vi "CheckingLimits.vi"(7 "References":T1, 10 "Limits":dbl[](array[numeric]), 11 "Data":dbl) -> (3 "Color":u32)   [LabVIEW 2019]
uses:
  TypeDef/#TypeDef_References.ctl
  TypeDef/#TypeDef_Buttons.ctl
  TypeDef/#TypeDef_ReferencesMeassurementProp.ctl
  TypeDef/#TypeDef_ReferencesArchiveProp.ctl
  TypeDef/#TypeDef_Lists.ctl
  TypeDef/#TypeDef_MeasProp.ctl
  TypeDef/#TypeDef_OpProp.ctl
  TypeDef/#TypeDef_Enum_ModeOp.ctl
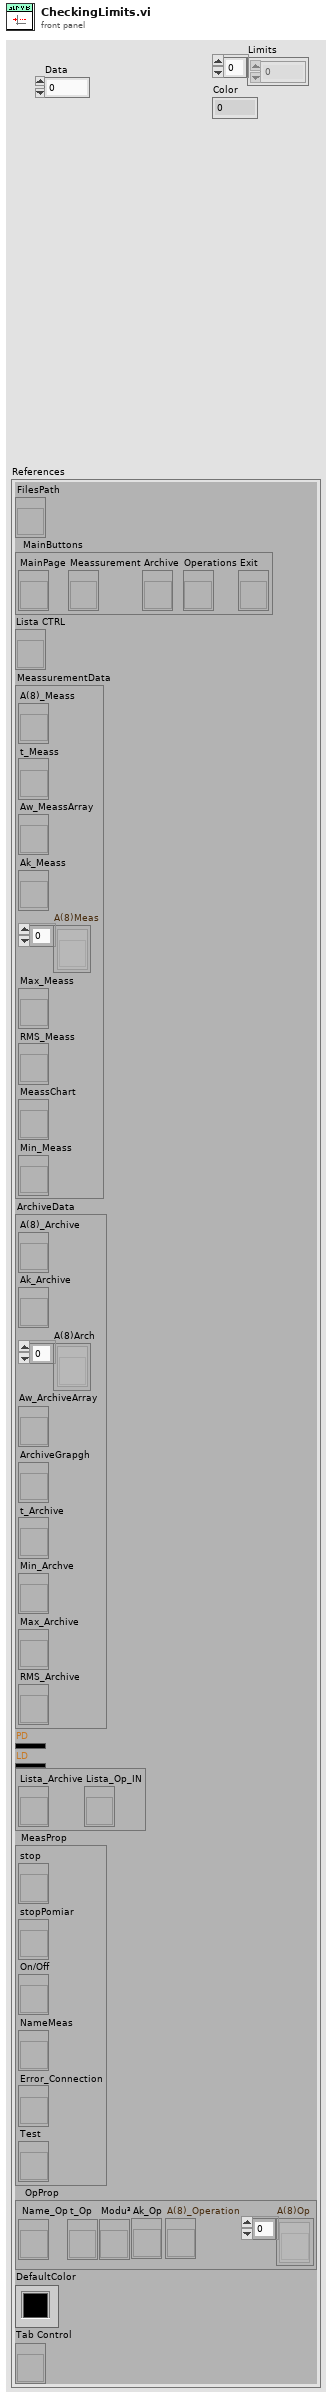
[diagram p1: front panel]
types:
  T1 = typedef "#TypeDef_References.ctl" = cluster{"FilesPath":refnum<vi>, "MainButtons":T2, "Lista CTRL":refnum<vi>, "MeassurementData":T3, "ArchiveData":T4, "PD":u32, "LD":u32, "Lists":T5, "MeasProp":T6, "OpProp":T7, "DefaultColor":u32, "Tab Control":refnum<vi>}
  T2 = typedef "#TypeDef_Buttons.ctl" = cluster{"MainPage":refnum<vi>, "Meassurement":refnum<vi>, "Archive":refnum<vi>, "Operations":refnum<vi>, "Exit":refnum<vi>}
  T3 = typedef "#TypeDef_ReferencesMeassurementProp.ctl" = cluster{"A(8)_Meass":refnum<vi>, "t_Meass":refnum<vi>, "Aw_MeassArray":refnum<vi>, "Ak_Meass":refnum<vi>, "A(8)Meas":refnum<vi>[], "Max_Meass":refnum<vi>, "RMS_Meass":refnum<vi>, "MeassChart":refnum<vi>, "Min_Meass":refnum<vi>}
  T4 = typedef "#TypeDef_ReferencesArchiveProp.ctl" = cluster{"A(8)_Archive":refnum<vi>, "Ak_Archive":refnum<vi>, "A(8)Arch":refnum<vi>[], "Aw_ArchiveArray":refnum<vi>, "ArchiveGrapgh":refnum<vi>, "t_Archive":refnum<vi>, "Min_Archve":refnum<vi>, "Max_Archive":refnum<vi>, "RMS_Archive":refnum<vi>}
  T5 = typedef "#TypeDef_Lists.ctl" = cluster{"Lista_Archive":refnum<vi>, "Lista_Op_IN":refnum<vi>}
  T6 = typedef "#TypeDef_MeasProp.ctl" = cluster{"stop":refnum<vi>, "stopPomiar":refnum<vi>, "On/Off":refnum<vi>, "NameMeas":refnum<vi>, "Error_Connection":refnum<vi>, "Test":refnum<vi>}
  T7 = typedef "#TypeDef_OpProp.ctl" = cluster{"Name_Op":refnum<vi>, "t_Op":refnum<vi>, "Modu³":refnum<vi>, "Ak_Op":refnum<vi>, "A(8)_Operation":refnum<vi>, "A(8)Op":refnum<vi>[]}
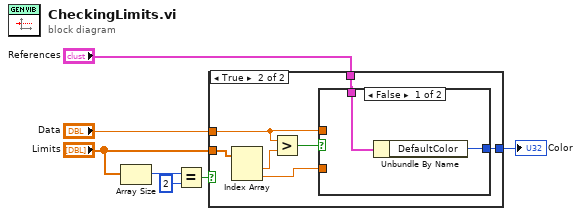
[diagram p0: block diagram]
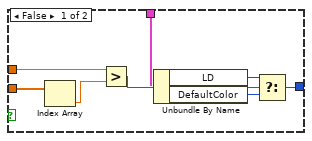
[diagram p2: hidden frame]
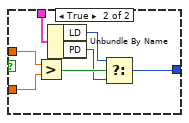
[diagram p3: hidden frame]
diagram:
  n1 = Array Size(array="Limits") -> (size(s)=w5:i32)
  n2 = Equal?(x=w5, y=2) -> (x = y?=w3:bool)
  n3 = case shown="True" w3 {
    tunnel: [w11 w22] -> w1
    tunnel: "Data" -> [w15 w19]
    tunnel: "Limits" -> [w13 w17]
    tunnel: "References" -> [w10 w16]
    frame False {
      n4 = Index Array(array=w13) -> (element=w14:dbl)  [unwired: 1 in]
      n5 = Greater?(x=w15, y=w14) -> (0:w12:bool)
      n6 = Unbundle By Name(w10) -> ("LD"=w9:u32, "DefaultColor"=w8:u32)
      n7 = Select(t=w9, s=w12, f=w8) -> (s? t:f=w11:u32)
    }
    frame True {
      n8 = Index Array(array=w17) -> (element #1=w20:dbl, element #2=w21:dbl)  [unwired: 2 in]
      n9 = Greater?(x=w19, y=w20) -> (0:w18:bool)
      n10 = case shown="False" w18 {
        tunnel: w19 -> [_ w31]
        tunnel: w21 -> [_ w30]
        tunnel: [w23 w28] -> w22
        tunnel: w16 -> [w24 w27]
        frame False {
          n11 = Unbundle By Name(w24) -> ("DefaultColor"=w23:u32)
        }
        frame True {
          n12 = Greater?(x=w31, y=w30) -> (0:w29:bool)
          n13 = Unbundle By Name(w27) -> ("LD"=w26:u32, "PD"=w25:u32)
          n14 = Select(t=w26, s=w29, f=w25) -> (s? t:f=w28:u32)
        }
      }
    }
  }
  "Color" <- w1
